vi "UI Initialize.vi"(8 "error in (no error)":errorcluster, 11 "UI ActorTop in":refnum<class "MCLB_Template.lvclass">) -> (0 "error out":errorcluster, 3 "UI ActorTop out":refnum<class "MCLB_Template.lvclass">)   [LabVIEW 2021, in "MCLB_Template.lvclass"]
doc: "UI: Initialize\n2015-03-18 16:27:22\n蒋松\njiangsong@outlook.com"
uses:
  MCLB_Template.lvclass
  <userlib>/John_Lib/AbstractActorTemplate/AbstractActorTemplate/UIActorTop.lvclass
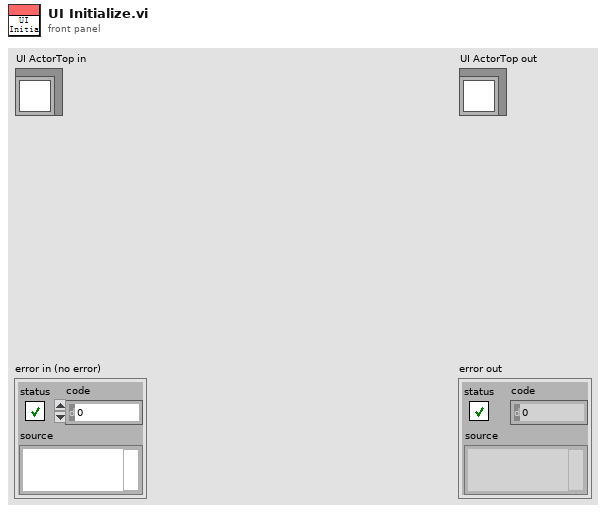
[diagram p1: front panel]
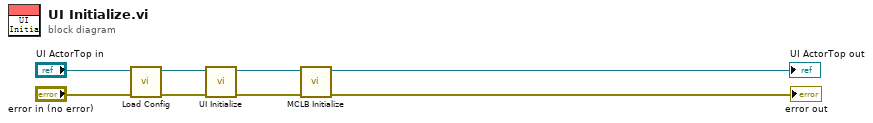
[diagram p0: block diagram]
diagram:
  n1 = call "Load Config.vi"("error in (no error)"="error in (no error)", "MCLB_Template in"="UI ActorTop in") -> ("error out"=w6:errorcluster, "MCLB_Template out"=w7:refnum<class "MCLB_Template.lvclass">)  [unwired: 8 in]
  n2 = call-parent "UI Initialize.vi"("error in (no error)"=w6, "UI ActorTop in"=w7) -> ("error out"=w2:errorcluster, "UI ActorTop out"=w4:refnum<class "MCLB_Template.lvclass">)  [unwired: 8 in]
  n3 = call "MCLB Initialize.vi"("error in (no error)"=w2, "MCLB_Template in"=w4) -> ("error out"=→"error out":errorcluster, "MCLB_Template out"=→"UI ActorTop out":refnum<class "MCLB_Template.lvclass">)  [unwired: 8 in]
